vi "Launch Subordinate Object.vi"(8 "error in (no error)":errorcluster, 9 "Name":string, 10 "Subordinate Object":refnum<class "Template Module.lvclass">, 11 "Measure Object in":refnum<class "Application Controller.lvclass">) -> (0 "error out":errorcluster, 2 "Nested Actor's Enqueuer":refnum<class "Message Enqueuer.lvclass">, 3 "Measure Object out":refnum<class "Application Controller.lvclass">)   [LabVIEW 2018, in "Application Controller.lvclass"]
uses:
  Application Controller.lvclass
  C:/github/LabActor/Worker/Worker.lvclass
  Template Module/Template Module.lvclass
  <vilib>/ActorFramework/Message Enqueuer/Message Enqueuer.lvclass
  Worker/Worker.lvclass
  C:/github/LabActor/Template Module/Template Module.lvclass
  45487106-d2ca-4a74-ad91-6f1a5ef0fa32.vi
  <vilib>/Utility/error.llb/Clear Errors.vi
  <vilib>/Utility/error.llb/Error Cluster From Error Code.vi
  <vilib>/ErrorRing/Error Ring.xnode
  Process Controller/Process Controller.lvclass
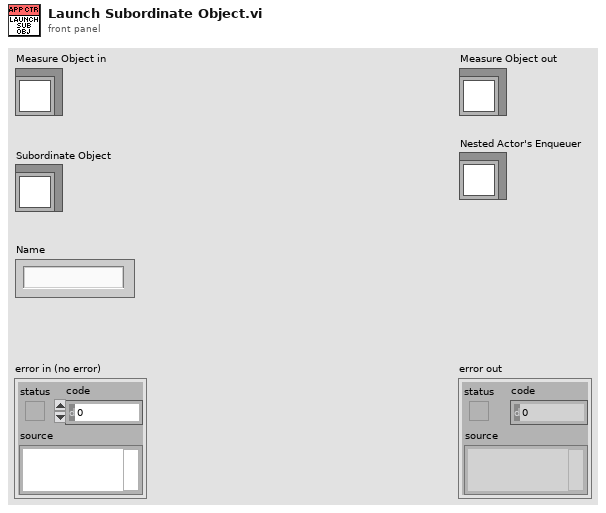
[diagram p1: front panel]
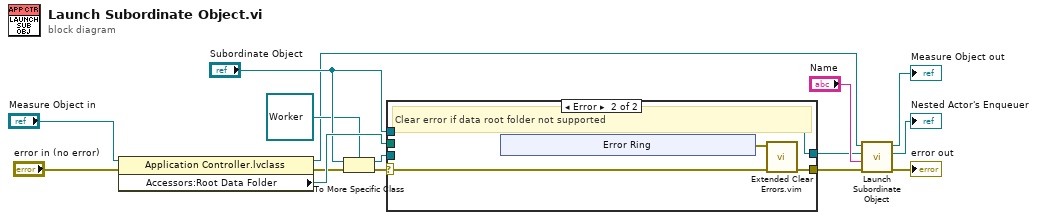
[diagram p0: block diagram]
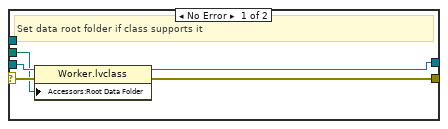
[diagram p2: hidden frame]
diagram:
  n1 = property class="Application Controller.lvclass"(reference="Measure Object in", error in="error in (no error)") -> (reference out=w1:refnum<class "Application Controller.lvclass">, error out=w7:errorcluster, "Accessors:Root Data Folder"=w8:path)
  n2 = To More Specific Class(target class=refnum<class "Worker.lvclass"> refnum ("Worker.lvclass"), reference="Subordinate Object", error in=w7) -> (specific class reference=w9:refnum<class "Worker.lvclass">, error out=w10:errorcluster)
  n3 = case shown="Error" w10 {
    selector: w10 -> [w20 w23]
    tunnel: w9 -> [w19 _]
    tunnel: w8 -> [w18 _]
    tunnel: [w17 w22] -> w6
    tunnel: [w16 w21] -> w5
    tunnel: "Subordinate Object" -> [_ w21]
    frame No Error {
      # "Set data root folder if class supports it"
      n4 = property class="Worker.lvclass"(reference=w19, error in=w20, "Accessors:Root Data Folder"=w18) -> (reference out=w16:refnum<class "Worker.lvclass">, error out=w17:errorcluster)
    }
    frame Error {
      # "Clear error if data root folder not supported"
      n5 = xnode "Error Ring"() -> ("error out"=w24:errorcluster)
      n6 = call "Extended Clear Errors.vim"("Error In"=w23, "specific error code to clear (0: all)"=w24) -> ("Error Out"=w22:errorcluster)  [unwired: 7 in, 2 out]
    }
  }
  n7 = call-parent "Launch Subordinate Object.vi"("error in (no error)"=w6, "Name"="Name", "Subordinate Object"=w5, "Template Module in"=w1) -> ("error out"=→"error out":errorcluster, "Nested Actor's Enqueuer"=→"Nested Actor's Enqueuer":refnum<class "Message Enqueuer.lvclass">, "Template Module out"=→"Measure Object out":refnum<class "Application Controller.lvclass">)  [unwired: 5 in]
